vi "9205_9206 32Ch Analog Input.vi"(1 "9205/6 I/O":T1={"9205/6 AI0"="NI 9205/AI0", "9205/6 AI1"="NI 9205/AI1", "9205/6 AI2"="NI 9205/AI2", "9205/6 AI3"="NI 9205/AI3", "9205/6 AI4"="NI 9205/AI4", "9205/6 AI5"="NI 9205/AI5", "9205/6 AI6"="NI 9205/AI6", "9205/6 AI7"="NI 9205/AI7", "9205/6 AI8"="NI 9205/AI8", "9205/6 AI9"="NI 9205/AI9", "9205/6 AI10"="NI 9205/AI10", "9205/6 AI11"="NI 9205/AI11", "9205/6 AI12"="NI 9205/AI12", "9205/6 AI13"="NI 9205/AI13", "9205/6 AI14"="NI 9205/AI14", "9205/6 AI15"="NI 9205/AI15", "9205/6 AI16"="NI 9205/AI16", "9205/6 AI17"="NI 9205/AI17", "9205/6 AI18"="NI 9205/AI18", "9205/6 AI19"="NI 9205/AI19", "9205/6 AI20"="NI 9205/AI20", "9205/6 AI21"="NI 9205/AI21", "9205/6 AI22"="NI 9205/AI22", "9205/6 AI23"="NI 9205/AI23", "9205/6 AI24"="NI 9205/AI24", "9205/6 AI25"="NI 9205/AI25", "9205/6 AI26"="NI 9205/AI26", "9205/6 AI27"="NI 9205/AI27", "9205/6 AI28"="NI 9205/AI28", "9205/6 AI29"="NI 9205/AI29", "9205/6 AI30"="NI 9205/AI30", "9205/6 AI31"="NI 9205/AI31"}) -> (0 "Packets":u64[](array[numeric]))   [LabVIEW 2009]
uses:
  <vilib>/eio/EIONode/EIONode.xnode
  <vilib>/rvi/eio/nirviEIOImplementation/nirviEIOImplementation.xnode
  <vilib>/rvi/eio/common/nirviEmuTemplateMethod_noerrors.vi
  <vilib>/rvi/eio/common/nirviEmuClasses.ctl
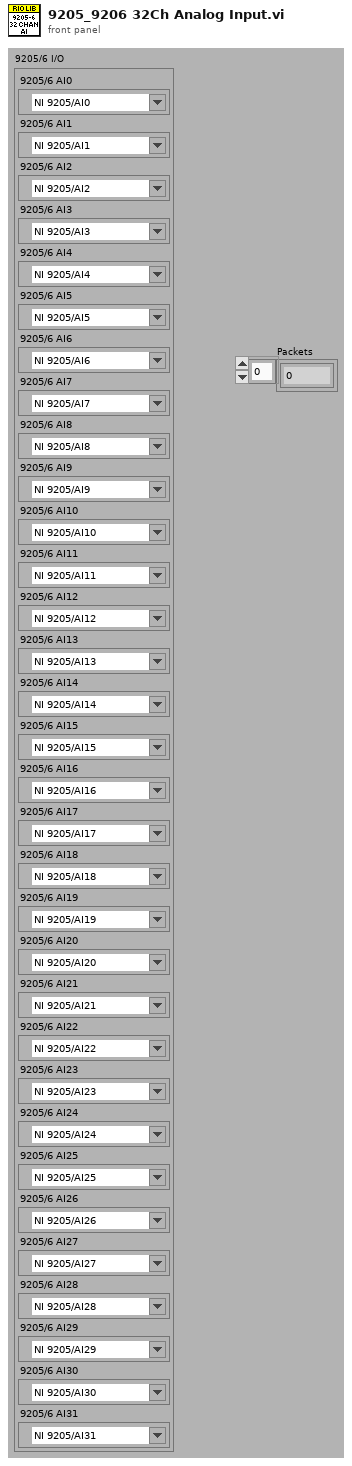
[diagram p1: front panel]
types:
  T1 = cluster{"9205/6 AI0":refnum<k21>, "9205/6 AI1":refnum<k21>, "9205/6 AI2":refnum<k21>, "9205/6 AI3":refnum<k21>, "9205/6 AI4":refnum<k21>, "9205/6 AI5":refnum<k21>, "9205/6 AI6":refnum<k21>, "9205/6 AI7":refnum<k21>, "9205/6 AI8":refnum<k21>, "9205/6 AI9":refnum<k21>, "9205/6 AI10":refnum<k21>, "9205/6 AI11":refnum<k21>, "9205/6 AI12":refnum<k21>, "9205/6 AI13":refnum<k21>, "9205/6 AI14":refnum<k21>, "9205/6 AI15":refnum<k21>, "9205/6 AI16":refnum<k21>, "9205/6 AI17":refnum<k21>, "9205/6 AI18":refnum<k21>, "9205/6 AI19":refnum<k21>, "9205/6 AI20":refnum<k21>, "9205/6 AI21":refnum<k21>, "9205/6 AI22":refnum<k21>, "9205/6 AI23":refnum<k21>, "9205/6 AI24":refnum<k21>, "9205/6 AI25":refnum<k21>, "9205/6 AI26":refnum<k21>, "9205/6 AI27":refnum<k21>, "9205/6 AI28":refnum<k21>, "9205/6 AI29":refnum<k21>, "9205/6 AI30":refnum<k21>, "9205/6 AI31":refnum<k21>}
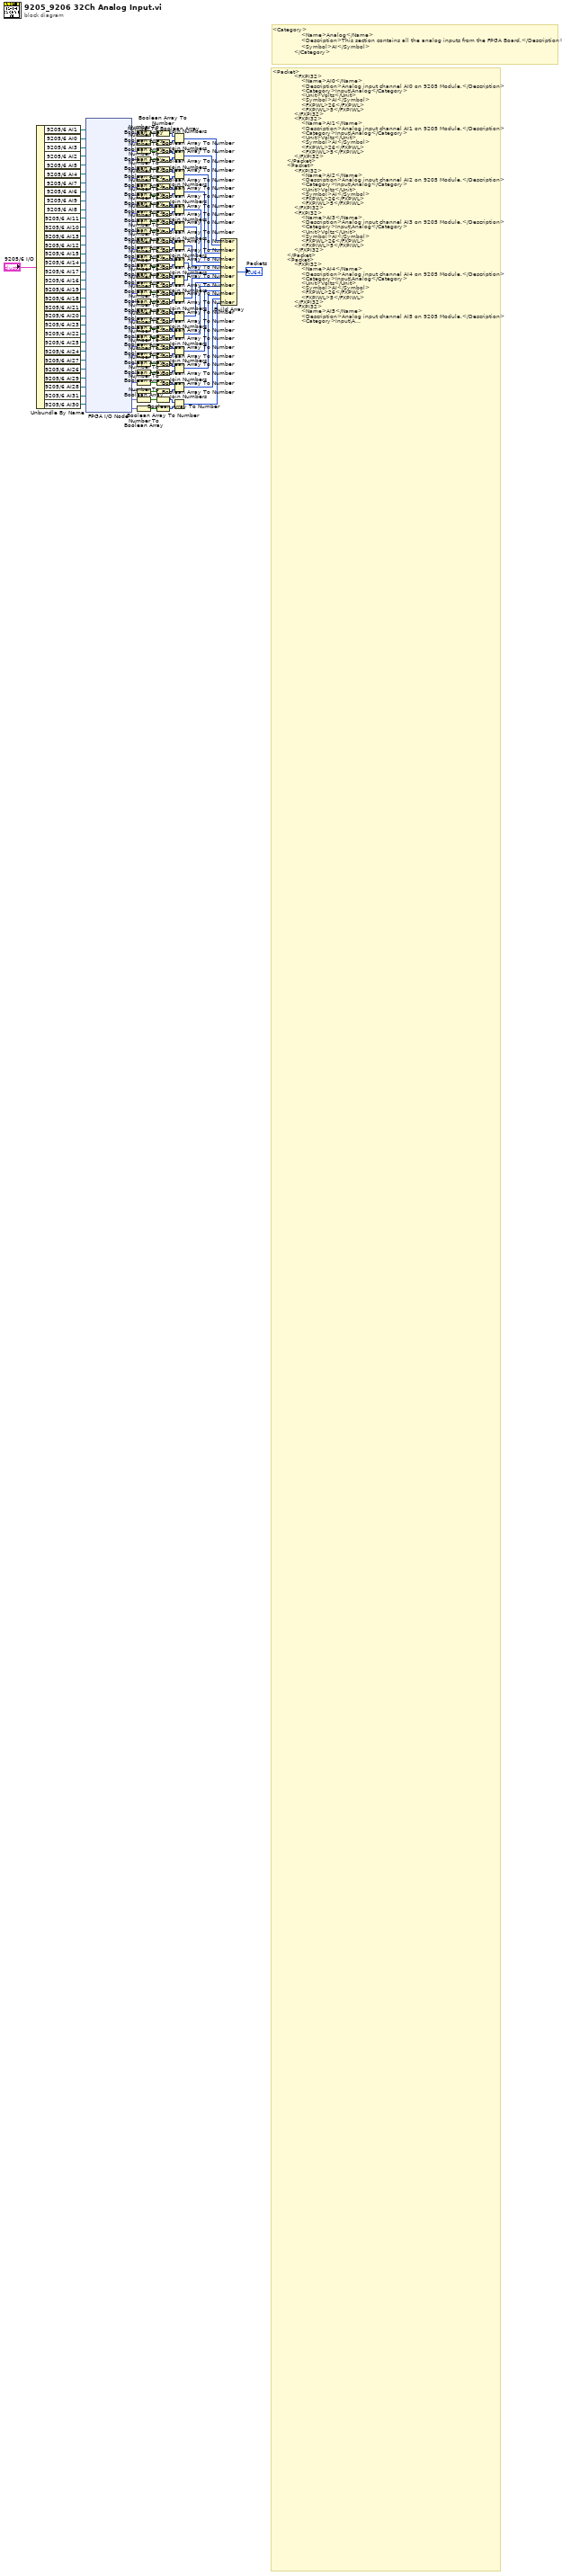
[diagram p0: block diagram]
diagram:
  # "<Category>\n                <Name>Analog</Name>\n                <Description>This section contains all the analog inputs from the FPGA Board.</Description>\n                <Symbol>AI</Symbol>\n            </Category>"
  # "<Packet>\n            <FXPI32>\n                <Name>AI0</Name>\n                <Description>Analog input channel AI0 on 9205 Module.</Description>\n                <Category>Input\\Analog</Category>\n                <Unit>Volts</Unit>\n                <Symbol>AI</Symbol>\n                <FXPWL>26</FXPWL>\n                <FXPIWL>5</FXPIWL>\n            </FXPI32>\n            <FXPI32>\n                <Name>AI1</Name>\n                <Description>Analog input channel AI1 on 9205 Module.</Description>\n                <Category>Input\\Analog</Category>\n                <Unit>Volts</Unit>\n                <Symbol>AI</Symbol>\n                <FXPWL>26</FXPWL>\n                <FXPIWL>5</FXPIWL>\n            </FXPI32>\n        </Packet>\n        <Packet>\n            <FXPI32>\n                <Name>AI2</Name>\n                <Description>Analog input channel AI2 on 9205 Module.</Description>\n                <Category>Input\\Analog</Category>\n                <Unit>Volts</Unit>\n                <Symbol>AI</Symbol>\n                <FXPWL>26</FXPWL>\n                <FXPIWL>5</FXPIWL>\n            </FXPI32>\n            <FXPI32>\n                <Name>AI3</Name>\n                <Description>Analog input channel AI3 on 9205 Module.</Description>\n                <Category>Input\\Analog</Category>\n                <Unit>Volts</Unit>\n                <Symbol>AI</Symbol>\n                <FXPWL>26</FXPWL>\n                <FXPIWL>5</FXPIWL>\n            </FXPI32>\n        </Packet>\n        <Packet>\n            <FXPI32>\n                <Name>AI4</Name>\n                <Description>Analog input channel AI4 on 9205 Module.</Description>\n                <Category>Input\\Analog</Category>\n                <Unit>Volts</Unit>\n                <Symbol>AI</Symbol>\n                <FXPWL>26</FXPWL>\n                <FXPIWL>5</FXPIWL>\n            </FXPI32>\n            <FXPI32>\n                <Name>AI5</Name>\n                <Description>Analog input channel AI5 on 9205 Module.</Description>\n                <Category>Input\\Analog</Category>\n                <Unit>Volts</Unit>\n                <Symbol>AI</Symbol>\n                <FXPWL>26</FXPWL>\n                <FXPIWL>5</FXPIWL>\n            </FXPI32>\n        </Packet>\n        <Packet>\n            <FXPI32>\n                <Name>AI6</Name>\n                <Description>Analog input channel AI6 on 9205 Module.</Description>\n                <Category>Input\\Analog</Category>\n                <Unit>Volts</Unit>\n                <Symbol>AI</Symbol>\n                <FXPWL>26</FXPWL>\n                <FXPIWL>5</FXPIWL>\n            </FXPI32>\n            <FXPI32>\n                <Name>AI7</Name>\n                <Description>Analog input channel AI7 on 9205 Module.</Description>\n                <Category>Input\\Analog</Category>\n                <Unit>Volts</Unit>\n                <Symbol>AI</Symbol>\n                <FXPWL>26</FXPWL>\n                <FXPIWL>5</FXPIWL>\n            </FXPI32>\n        </Packet>\n        <Packet>\n            <FXPI32>\n                <Name>AI8</Name>\n                <Description>Analog input channel AI8 on 9205 Module.</Description>\n                <Category>Input\\Analog</Category>\n                <Unit>Volts</Unit>\n                <Symbol>AI</Symbol>\n                <FXPWL>26</FXPWL>\n                <FXPIWL>5</FXPIWL>\n            </FXPI32>\n            <FXPI32>\n                <Name>AI9</Name>\n                <Description>Analog input channel AI9 on 9205 Module.</Description>\n                <Category>Input\\Analog</Category>\n                <Unit>Volts</Unit>\n                <Symbol>AI</Symbol>\n                <FXPWL>26</FXPWL>\n                <FXPIWL>5</FXPIWL>\n            </FXPI32>\n        </Packet>\n        <Packet>\n            <FXPI32>\n                <Name>AI10</Name>\n                <Description>Analog input channel AI10 on 9205 Module.</Description>\n                <Category>Input\\Analog</Category>\n                <Unit>Volts</Unit>\n                <Symbol>AI</Symbol>\n                <FXPWL>26</FXPWL>\n                <FXPIWL>5</FXPIWL>\n            </FXPI32>\n            <FXPI32>\n                <Name>AI11</Name>\n                <Description>Analog input channel AI11 on 9205 Module.</Description>\n                <Category>Input\\Analog</Category>\n                <Unit>Volts</Unit>\n                <Symbol>AI</Symbol>\n                <FXPWL>26</FXPWL>\n                <FXPIWL>5</FXPIWL>\n            </FXPI32>\n        </Packet>\n        <Packet>\n            <FXPI32>\n                <Name>AI12</Name>\n                <Description>Analog input channel AI12 on 9205 Module.</Description>\n                <Category>Input\\Analog</Category>\n                <Unit>Volts</Unit>\n                <Symbol>AI</Symbol>\n                <FXPWL>26</FXPWL>\n                <FXPIWL>5</FXPIWL>\n            </FXPI32>\n            <FXPI32>\n                <Name>AI13</Name>\n                <Description>Analog input channel AI13 on 9205 Module.</Description>\n                <Category>Input\\Analog</Category>\n                <Unit>Volts</Unit>\n                <Symbol>AI</Symbol>\n                <FXPWL>26</FXPWL>\n                <FXPIWL>5</FXPIWL>\n            </FXPI32>\n        </Packet>\n        <Packet>\n            <FXPI32>\n                <Name>AI14</Name>\n                <Description>Analog input channel AI14 on 9205 Module.</Description>\n                <Category>Input\\Analog</Category>\n                <Unit>Volts</Unit>\n                <Symbol>AI</Symbol>\n                <FXPWL>26</FXPWL>\n                <FXPIWL>5</FXPIWL>\n            </FXPI32>\n            <FXPI32>\n                <Name>AI15</Name>\n                <Description>Analog input channel AI15 on 9205 Module.</Description>\n                <Category>Input\\Analog</Category>\n                <Unit>Volts</Unit>\n                <Symbol>AI</Symbol>\n                <FXPWL>26</FXPWL>\n                <FXPIWL>5</FXPIWL>\n            </FXPI32>\n        </Packet>\n        <Packet>\n            <FXPI32>\n                <Name>AI16</Name>\n                <Description>Analog input channel AI16 on 9205 Module.</Description>\n                <Category>Input\\Analog</Category>\n                <Unit>Volts</Unit>\n                <Symbol>AI</Symbol>\n                <FXPWL>26</FXPWL>\n                <FXPIWL>5</FXPIWL>\n            </FXPI32>\n            <FXPI32>\n                <Name>AI17</Name>\n                <Description>Analog input channel AI17 on 9205 Module.</Description>\n                <Category>Input\\Analog</Category>\n                <Unit>Volts</Unit>\n                <Symbol>AI</Symbol>\n                <FXPWL>26</FXPWL>\n                <FXPIWL>5</FXPIWL>\n            </FXPI32>\n        </Packet>\n        <Packet>\n            <FXPI32>\n                <Name>AI18</Name>\n                <Description>Analog input channel AI18 on 9205 Module.</Description>\n                <Category>Input\\Analog</Category>\n                <Unit>Volts</Unit>\n                <Symbol>AI</Symbol>\n                <FXPWL>26</FXPWL>\n                <FXPIWL>5</FXPIWL>\n            </FXPI32>\n            <FXPI32>\n                <Name>AI19</Name>\n                <Description>Analog input channel AI19 on 9205 Module.</Description>\n                <Category>Input\\Analog</Category>\n                <Unit>Volts</Unit>\n                <Symbol>AI</Symbol>\n                <FXPWL>26</FXPWL>\n                <FXPIWL>5</FXPIWL>\n            </FXPI32>\n        </Packet>\n        <Packet>\n            <FXPI32>\n                <Name>AI20</Name>\n                <Description>Analog input channel AI20 on 9205 Module.</Description>\n                <Category>Input\\Analog</Category>\n                <Unit>Volts</Unit>\n                <Symbol>AI</Symbol>\n                <FXPWL>26</FXPWL>\n                <FXPIWL>5</FXPIWL>\n            </FXPI32>\n            <FXPI32>\n                <Name>AI21</Name>\n                <Description>Analog input channel AI21 on 9205 Module.</Description>\n                <Category>Input\\Analog</Category>\n                <Unit>Volts</Unit>\n                <Symbol>AI</Symbol>\n                <FXPWL>26</FXPWL>\n                <FXPIWL>5</FXPIWL>\n            </FXPI32>\n        </Packet>\n        <Packet>\n            <FXPI32>\n                <Name>AI22</Name>\n                <Description>Analog input channel AI22 on 9205 Module.</Description>\n                <Category>Input\\Analog</Category>\n                <Unit>Volts</Unit>\n                <Symbol>AI</Symbol>\n                <FXPWL>26</FXPWL>\n                <FXPIWL>5</FXPIWL>\n            </FXPI32>\n            <FXPI32>\n                <Name>AI23</Name>\n                <Description>Analog input channel AI23 on 9205 Module.</Description>\n                <Category>Input\\Analog</Category>\n                <Unit>Volts</Unit>\n                <Symbol>AI</Symbol>\n                <FXPWL>26</FXPWL>\n                <FXPIWL>5</FXPIWL>\n            </FXPI32>\n        </Packet>\n        <Packet>\n            <FXPI32>\n                <Name>AI24</Name>\n                <Description>Analog input channel AI24 on 9205 Module.</Description>\n                <Category>Input\\Analog</Category>\n                <Unit>Volts</Unit>\n                <Symbol>AI</Symbol>\n                <FXPWL>26</FXPWL>\n                <FXPIWL>5</FXPIWL>\n            </FXPI32>\n            <FXPI32>\n                <Name>AI25</Name>\n                <Description>Analog input channel AI25 on 9205 Module.</Description>\n                <Category>Input\\Analog</Category>\n                <Unit>Volts</Unit>\n                <Symbol>AI</Symbol>\n                <FXPWL>26</FXPWL>\n                <FXPIWL>5</FXPIWL>\n            </FXPI32>\n        </Packet>\n        <Packet>\n            <FXPI32>\n                <Name>AI26</Name>\n                <Description>Analog input channel AI26 on 9205 Module.</Description>\n                <Category>Input\\Analog</Category>\n                <Unit>Volts</Unit>\n                <Symbol>AI</Symbol>\n                <FXPWL>26</FXPWL>\n                <FXPIWL>5</FXPIWL>\n            </FXPI32>\n            <FXPI32>\n                <Name>AI27</Name>\n                <Description>Analog input channel AI27 on 9205 Module.</Description>\n                <Category>Input\\Analog</Category>\n                <Unit>Volts</Unit>\n                <Symbol>AI</Symbol>\n                <FXPWL>26</FXPWL>\n                <FXPIWL>5</FXPIWL>\n            </FXPI32>\n        </Packet>\n        <Packet>\n            <FXPI32>\n                <Name>AI28</Name>\n                <Description>Analog input channel AI28 on 9205 Module.</Description>\n                <Category>Input\\Analog</Category>\n                <Unit>Volts</Unit>\n                <Symbol>AI</Symbol>\n                <FXPWL>26</FXPWL>\n                <FXPIWL>5</FXPIWL>\n            </FXPI32>\n            <FXPI32>\n                <Name>AI29</Name>\n                <Description>Analog input channel AI29 on 9205 Module.</Description>\n                <Category>Input\\Analog</Category>\n                <Unit>Volts</Unit>\n                <Symbol>AI</Symbol>\n                <FXPWL>26</FXPWL>\n                <FXPIWL>5</FXPIWL>\n            </FXPI32>\n        </Packet>\n        <Packet>\n            <FXPI32>\n                <Name>AI30</Name>\n                <Description>Analog input channel AI30 on 9205 Module.</Description>\n                <Category>Input\\Analog</Category>\n                <Unit>Volts</Unit>\n                <Symbol>AI</Symbol>\n                <FXPWL>26</FXPWL>\n                <FXPIWL>5</FXPIWL>\n            </FXPI32>\n            <FXPI32>\n                <Name>AI31</Name>\n                <Description>Analog input channel AI31 on 9205 Module.</Description>\n                <Category>Input\\Analog</Category>\n                <Unit>Volts</Unit>\n                <Symbol>AI</Symbol>\n                <FXPWL>26</FXPWL>\n                <FXPIWL>5</FXPIWL>\n            </FXPI32>\n        </Packet>"
  n1 = Unbundle By Name("9205/6 I/O") -> ("9205/6 AI1"=w127:refnum<k21>, "9205/6 AI0"=w130:refnum<k21>, "9205/6 AI3"=w128:refnum<k21>, "9205/6 AI2"=w131:refnum<k21>, "9205/6 AI5"=w123:refnum<k21>, "9205/6 AI4"=w124:refnum<k21>, "9205/6 AI7"=w125:refnum<k21>, "9205/6 AI6"=w126:refnum<k21>, "9205/6 AI9"=w108:refnum<k21>, "9205/6 AI8"=w107:refnum<k21>, "9205/6 AI11"=w106:refnum<k21>, "9205/6 AI10"=w105:refnum<k21>, "9205/6 AI13"=w104:refnum<k21>, "9205/6 AI12"=w103:refnum<k21>, "9205/6 AI15"=w102:refnum<k21>, "9205/6 AI14"=w101:refnum<k21>, "9205/6 AI17"=w72:refnum<k21>, "9205/6 AI16"=w71:refnum<k21>, "9205/6 AI19"=w70:refnum<k21>, "9205/6 AI18"=w69:refnum<k21>, "9205/6 AI21"=w68:refnum<k21>, "9205/6 AI20"=w67:refnum<k21>, "9205/6 AI23"=w66:refnum<k21>, "9205/6 AI22"=w65:refnum<k21>, "9205/6 AI25"=w64:refnum<k21>, "9205/6 AI24"=w63:refnum<k21>, "9205/6 AI27"=w57:refnum<k21>, "9205/6 AI26"=w58:refnum<k21>, "9205/6 AI29"=w59:refnum<k21>, "9205/6 AI28"=w60:refnum<k21>, "9205/6 AI31"=w61:refnum<k21>, "9205/6 AI30"=w62:refnum<k21>)
  n2 = xnode "FPGA I/O Node"("FPGA I/O In"=w127, "FPGA I/O In"=w130, "FPGA I/O In"=w128, "FPGA I/O In"=w131, "FPGA I/O In"=w123, "FPGA I/O In"=w124, "FPGA I/O In"=w125, "FPGA I/O In"=w126, "FPGA I/O In"=w108, "FPGA I/O In"=w107, "FPGA I/O In"=w106, "FPGA I/O In"=w105, "FPGA I/O In"=w104, "FPGA I/O In"=w103, "FPGA I/O In"=w102, "FPGA I/O In"=w101, "FPGA I/O In"=w72, "FPGA I/O In"=w71, "FPGA I/O In"=w70, "FPGA I/O In"=w69, "FPGA I/O In"=w68, "FPGA I/O In"=w67, "FPGA I/O In"=w66, "FPGA I/O In"=w65, "FPGA I/O In"=w64, "FPGA I/O In"=w63, "FPGA I/O In"=w57, "FPGA I/O In"=w58, "FPGA I/O In"=w59, "FPGA I/O In"=w60, "FPGA I/O In"=w61, "FPGA I/O In"=w62) -> ("I/O Item"=w137:fxp<+/-,26,5>, "I/O Item"=w139:fxp<+/-,26,5>, "I/O Item"=w129:fxp<+/-,26,5>, "I/O Item"=w138:fxp<+/-,26,5>, "I/O Item"=w111:fxp<+/-,26,5>, "I/O Item"=w112:fxp<+/-,26,5>, "I/O Item"=w113:fxp<+/-,26,5>, "I/O Item"=w114:fxp<+/-,26,5>, "I/O Item"=w84:fxp<+/-,26,5>, "I/O Item"=w83:fxp<+/-,26,5>, "I/O Item"=w82:fxp<+/-,26,5>, "I/O Item"=w81:fxp<+/-,26,5>, "I/O Item"=w80:fxp<+/-,26,5>, "I/O Item"=w79:fxp<+/-,26,5>, "I/O Item"=w78:fxp<+/-,26,5>, "I/O Item"=w77:fxp<+/-,26,5>, "I/O Item"=w24:fxp<+/-,26,5>, "I/O Item"=w9:fxp<+/-,26,5>, "I/O Item"=w10:fxp<+/-,26,5>, "I/O Item"=w11:fxp<+/-,26,5>, "I/O Item"=w12:fxp<+/-,26,5>, "I/O Item"=w13:fxp<+/-,26,5>, "I/O Item"=w14:fxp<+/-,26,5>, "I/O Item"=w15:fxp<+/-,26,5>, "I/O Item"=w16:fxp<+/-,26,5>, "I/O Item"=w17:fxp<+/-,26,5>, "I/O Item"=w18:fxp<+/-,26,5>, "I/O Item"=w19:fxp<+/-,26,5>, "I/O Item"=w20:fxp<+/-,26,5>, "I/O Item"=w21:fxp<+/-,26,5>, "I/O Item"=w22:fxp<+/-,26,5>, "I/O Item"=w23:fxp<+/-,26,5>)  [unwired: 32 out]
  n3 = Number To Boolean Array(number=w137) -> (Boolean array=w133:bool[])
  n4 = Number To Boolean Array(number=w139) -> (Boolean array=w134:bool[])
  n5 = Number To Boolean Array(number=w129) -> (Boolean array=w136:bool[])
  n6 = Number To Boolean Array(number=w138) -> (Boolean array=w135:bool[])
  n7 = Number To Boolean Array(number=w111) -> (Boolean array=w122:bool[])
  n8 = Number To Boolean Array(number=w112) -> (Boolean array=w121:bool[])
  n9 = Number To Boolean Array(number=w113) -> (Boolean array=w119:bool[])
  n10 = Number To Boolean Array(number=w114) -> (Boolean array=w120:bool[])
  n11 = Number To Boolean Array(number=w84) -> (Boolean array=w92:bool[])
  n12 = Number To Boolean Array(number=w83) -> (Boolean array=w91:bool[])
  n13 = Number To Boolean Array(number=w82) -> (Boolean array=w89:bool[])
  n14 = Number To Boolean Array(number=w81) -> (Boolean array=w90:bool[])
  n15 = Number To Boolean Array(number=w80) -> (Boolean array=w93:bool[])
  n16 = Number To Boolean Array(number=w79) -> (Boolean array=w94:bool[])
  n17 = Number To Boolean Array(number=w78) -> (Boolean array=w96:bool[])
  n18 = Number To Boolean Array(number=w77) -> (Boolean array=w95:bool[])
  n19 = Number To Boolean Array(number=w24) -> (Boolean array=w32:bool[])
  n20 = Number To Boolean Array(number=w9) -> (Boolean array=w31:bool[])
  n21 = Number To Boolean Array(number=w10) -> (Boolean array=w29:bool[])
  n22 = Number To Boolean Array(number=w11) -> (Boolean array=w30:bool[])
  n23 = Number To Boolean Array(number=w12) -> (Boolean array=w33:bool[])
  n24 = Number To Boolean Array(number=w13) -> (Boolean array=w34:bool[])
  n25 = Number To Boolean Array(number=w14) -> (Boolean array=w36:bool[])
  n26 = Number To Boolean Array(number=w15) -> (Boolean array=w35:bool[])
  n27 = Number To Boolean Array(number=w16) -> (Boolean array=w49:bool[])
  n28 = Number To Boolean Array(number=w17) -> (Boolean array=w50:bool[])
  n29 = Number To Boolean Array(number=w18) -> (Boolean array=w52:bool[])
  n30 = Number To Boolean Array(number=w19) -> (Boolean array=w51:bool[])
  n31 = Number To Boolean Array(number=w20) -> (Boolean array=w48:bool[])
  n32 = Number To Boolean Array(number=w21) -> (Boolean array=w47:bool[])
  n33 = Number To Boolean Array(number=w22) -> (Boolean array=w45:bool[])
  n34 = Number To Boolean Array(number=w23) -> (Boolean array=w46:bool[])
  n35 = Boolean Array To Number(Boolean array=w133) -> (number=w140:u32)
  n36 = Boolean Array To Number(Boolean array=w134) -> (number=w141:u32)
  n37 = Boolean Array To Number(Boolean array=w136) -> (number=w142:u32)
  n38 = Boolean Array To Number(Boolean array=w135) -> (number=w143:u32)
  n39 = Boolean Array To Number(Boolean array=w122) -> (number=w118:u32)
  n40 = Boolean Array To Number(Boolean array=w121) -> (number=w117:u32)
  n41 = Boolean Array To Number(Boolean array=w119) -> (number=w116:u32)
  n42 = Boolean Array To Number(Boolean array=w120) -> (number=w115:u32)
  n43 = Boolean Array To Number(Boolean array=w92) -> (number=w88:u32)
  n44 = Boolean Array To Number(Boolean array=w91) -> (number=w87:u32)
  n45 = Boolean Array To Number(Boolean array=w89) -> (number=w86:u32)
  n46 = Boolean Array To Number(Boolean array=w90) -> (number=w85:u32)
  n47 = Boolean Array To Number(Boolean array=w93) -> (number=w97:u32)
  n48 = Boolean Array To Number(Boolean array=w94) -> (number=w98:u32)
  n49 = Boolean Array To Number(Boolean array=w96) -> (number=w99:u32)
  n50 = Boolean Array To Number(Boolean array=w95) -> (number=w100:u32)
  n51 = Boolean Array To Number(Boolean array=w32) -> (number=w28:u32)
  n52 = Boolean Array To Number(Boolean array=w31) -> (number=w27:u32)
  n53 = Boolean Array To Number(Boolean array=w29) -> (number=w26:u32)
  n54 = Boolean Array To Number(Boolean array=w30) -> (number=w25:u32)
  n55 = Boolean Array To Number(Boolean array=w33) -> (number=w37:u32)
  n56 = Boolean Array To Number(Boolean array=w34) -> (number=w38:u32)
  n57 = Boolean Array To Number(Boolean array=w36) -> (number=w39:u32)
  n58 = Boolean Array To Number(Boolean array=w35) -> (number=w40:u32)
  n59 = Boolean Array To Number(Boolean array=w49) -> (number=w53:u32)
  n60 = Boolean Array To Number(Boolean array=w50) -> (number=w54:u32)
  n61 = Boolean Array To Number(Boolean array=w52) -> (number=w55:u32)
  n62 = Boolean Array To Number(Boolean array=w51) -> (number=w56:u32)
  n63 = Boolean Array To Number(Boolean array=w48) -> (number=w44:u32)
  n64 = Boolean Array To Number(Boolean array=w47) -> (number=w43:u32)
  n65 = Boolean Array To Number(Boolean array=w45) -> (number=w42:u32)
  n66 = Boolean Array To Number(Boolean array=w46) -> (number=w41:u32)
  n67 = Join Numbers(hi=w140, lo=w141) -> ((hi.lo)=w144:u64)
  n68 = Join Numbers(hi=w118, lo=w117) -> ((hi.lo)=w109:u64)
  n69 = Join Numbers(hi=w88, lo=w87) -> ((hi.lo)=w73:u64)
  n70 = Join Numbers(hi=w97, lo=w98) -> ((hi.lo)=w75:u64)
  n71 = Join Numbers(hi=w28, lo=w27) -> ((hi.lo)=w2:u64)
  n72 = Join Numbers(hi=w37, lo=w38) -> ((hi.lo)=w4:u64)
  n73 = Join Numbers(hi=w53, lo=w54) -> ((hi.lo)=w1:u64)
  n74 = Join Numbers(hi=w44, lo=w43) -> ((hi.lo)=w7:u64)
  n75 = Join Numbers(hi=w142, lo=w143) -> ((hi.lo)=w145:u64)
  n76 = Join Numbers(hi=w116, lo=w115) -> ((hi.lo)=w110:u64)
  n77 = Join Numbers(hi=w86, lo=w85) -> ((hi.lo)=w74:u64)
  n78 = Join Numbers(hi=w99, lo=w100) -> ((hi.lo)=w76:u64)
  n79 = Join Numbers(hi=w26, lo=w25) -> ((hi.lo)=w3:u64)
  n80 = Join Numbers(hi=w39, lo=w40) -> ((hi.lo)=w5:u64)
  n81 = Join Numbers(hi=w55, lo=w56) -> ((hi.lo)=w6:u64)
  n82 = Join Numbers(hi=w42, lo=w41) -> ((hi.lo)=w8:u64)
  n83 = Build Array(w144, w145, w109, w110, w73, w74, w75, w76, w2, w3, w4, w5, w1, w6, w7, w8) -> (→"Packets":u64[])
